vi "Get Reference.vi"(11 "Init?":bool) -> (0 "error out":errorcluster, 3 "DVR":refnum<data-value>)   [LabVIEW 2012, in "Error Logger.lvclass"]
uses:
  Error Logger.lvclass
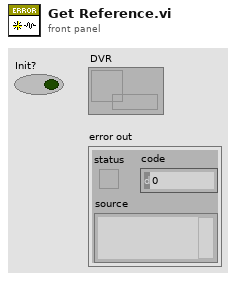
[diagram p1: front panel]
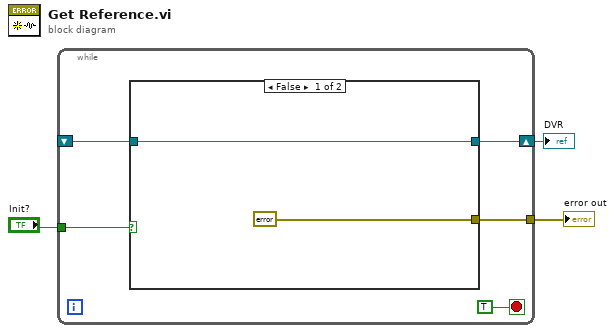
[diagram p0: block diagram]
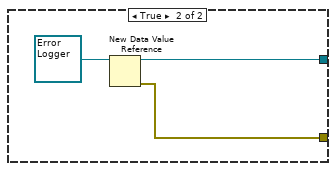
[diagram p2: hidden frame]
diagram:
  n1 = while {
    tunnel: "Init?" -> [w8]
    shift-right: [w7] -> w1
    shift-left: _ -> [w6]
    tunnel: [w4] -> w2
    stop <- TRUE stop-if-true
    n2 = case shown="False" w8 {
      tunnel: [w10 w12] -> w7
      tunnel: w6 -> [w10 _]
      tunnel: [errorcluster {"status"=FALSE, "code"=0, "source"=""} ("error out") w11] -> w4
      frame False {
      }
      frame True {
        n3 = New Data Value Reference(data value=refnum<class "Error Logger.lvclass"> refnum ("Error Logger out")) -> (data value reference=w12:refnum<data-value>, error out=w11:errorcluster)  [unwired: 1 in]
      }
    }
  }
  "error out" <- w2
  "DVR" <- w1
